vi "KE26XX Config Source & Measure.vi"(3 "Error Query (False)":bool, 4 "Limit":dbl=1.0, 5 "Measure Function (Current)":T1(ring), 6 "Level":dbl=1.0, 7 "Source Function (Current)":enum32{"Current", "Voltage"}(ring)=enum."Voltage", 8 "error in (no error)":errorcluster, 9 "Channel (Channel A)":T2, 10 "Node (0-64)":i8 min=0 max=64 step=1, 11 "VISA resource name":refnum<visa-resource-name>) -> (0 "error out":errorcluster, 1 "Output":string)   [LabVIEW 2018]
doc: "This example shows how to configure the source and take a measurement."
uses:
  <instrlib>/Keithley 2600 Series/Public/Channel.ctl
  <instrlib>/Keithley 2600 Series/Keithley 2600 Series.lvlib
panel:
  # "(c) 2008 Keithley Instruments, Inc.  ALL RIGHTS RESERVED."
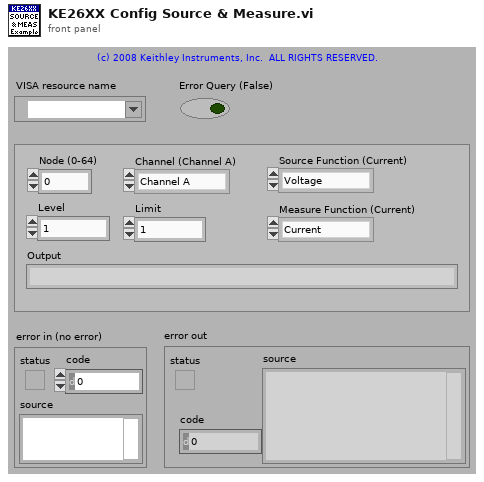
[diagram p1: front panel]
types:
  T1 = enum32{"Current", "Voltage", "IV", "Resistance", "Power"}
  T2 = typedef "Keithley 2600 Series.lvlib/Channel.ctl" = enum32{"Channel A", "Channel B"}
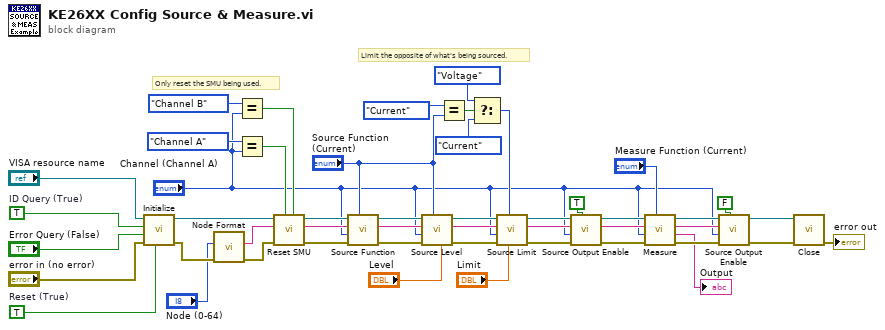
[diagram p0: block diagram]
diagram:
  w16 = TRUE  # Reset (True)
  w46 = TRUE  # ID Query (True)
  # "Limit the opposite of what's being sourced."
  # "Only reset the SMU being used."
  n1 = call <instrlib>:"Initialize.vi"("Reset (True)"=w16, "error in (no error)"="error in (no error)", "Error Query (False)"="Error Query (False)", "ID Query (True)"=w46, "VISA resource name"="VISA resource name") -> ("error out"=w5:errorcluster, "VISA resource name out"=w44:refnum<visa-resource-name>)  [unwired: 1 in, 4 out]
  n2 = call <instrlib>:"Node Format.vi"("error in"=w5, "Node (0-64)"="Node (0-64)") -> ("error out"=w4:errorcluster, "Formatted Node"=w6:string)  [unwired: 8 out]
  n3 = Equal?(x=enum32{"Channel A", "Channel B"}."Channel B", y="Channel (Channel A)") -> (x = y?=w40:bool)
  n4 = Equal?(x=enum32{"Channel A", "Channel B"}."Channel A", y="Channel (Channel A)") -> (x = y?=w41:bool)
  n5 = call <instrlib>:"Reset SMU.vi"("SMU B (No)"=w40, "SMU A (No)"=w41, "error in (no error)"=w4, "Node In"=w6, "VISA resource name"=w44) -> ("error out"=w39:errorcluster, "Node Out"=w37:string, "VISA resource name out"=w38:refnum<visa-resource-name>)  [unwired: 4 out]
  n6 = call <instrlib>:"Source Function.vi"("Function (Current)"="Source Function (Current)", "error in (no error)"=w39, "Channel (Channel A)"="Channel (Channel A)", "Node In"=w37, "VISA resource name"=w38) -> ("error out"=w34:errorcluster, "Node Out"=w36:string, "VISA resource name out"=w35:refnum<visa-resource-name>)  [unwired: 4 out]
  n7 = call <instrlib>:"Source Level.vi"("Level (0.000)"="Level", "Function (Current)"="Source Function (Current)", "error in (no error)"=w34, "Channel (Channel A)"="Channel (Channel A)", "Node In"=w36, "VISA resource name"=w35) -> ("error out"=w33:errorcluster, "Node Out"=w20:string, "VISA resource name out"=w32:refnum<visa-resource-name>)  [unwired: 3 out]
  n8 = Equal?(x=enum32{"Current", "Voltage"}."Current", y="Source Function (Current)") -> (x = y?=w13:bool)
  n9 = Select(t=enum32{"Current", "Voltage"}."Voltage" ("x"), s=w13, f=enum32{"Current", "Voltage"}."Current") -> (s? t:f=w11:enum32{"Current", "Voltage"})
  n10 = call <instrlib>:"Source Limit.vi"("Limit (0.000)"="Limit", "Function (Current)"=w11, "error in (no error)"=w33, "Channel (Channel A)"="Channel (Channel A)", "Node In"=w20, "VISA resource name"=w32) -> ("error out"=w30:errorcluster, "Node Out"=w19:string, "VISA resource name out"=w31:refnum<visa-resource-name>)  [unwired: 3 out]
  n11 = call <instrlib>:"Source Output Enable.vi"("Output (Off)"=TRUE, "error in (no error)"=w30, "Channel (Channel A)"="Channel (Channel A)", "Node In"=w19, "VISA resource name"=w31) -> ("error out"=w29:errorcluster, "Node Out"=w18:string, "VISA resource name out"=w28:refnum<visa-resource-name>)  [unwired: 4 out]
  n12 = call <instrlib>:"Measure.vi"("Function (Current)"="Measure Function (Current)", "error in (no error)"=w29, "Channel (Channel A)"="Channel (Channel A)", "Node In"=w18, "VISA resource name"=w28) -> ("error out"=w26:errorcluster, "Output"=→"Output":string, "Node Out"=w17:string, "VISA resource name out"=w27:refnum<visa-resource-name>)  [unwired: 2 in, 1 out]
  n13 = call <instrlib>:"Source Output Enable.vi"("Output (Off)"=FALSE, "error in (no error)"=w26, "Channel (Channel A)"="Channel (Channel A)", "Node In"=w17, "VISA resource name"=w27) -> ("error out"=w25:errorcluster, "VISA resource name out"=w24:refnum<visa-resource-name>)  [unwired: 5 out]
  n14 = call <instrlib>:"Close.vi"("error in (no error)"=w25, "VISA resource name"=w24) -> ("error out"=→"error out":errorcluster)  [unwired: 9 out]
